vi "Stop Core.vi"(10 "final error code":i32, 11 "Caller in":refnum<class "Caller.lvclass">) -> (3 "Caller out":refnum<class "Caller.lvclass">)   [LabVIEW 2020, in "Caller.lvlib" / "Caller.lvclass"]
doc: "(<B>Filename</B>: Actor Framework.lvlib:Actor.lvclass:Stop Core.vi)\n\nDefines what the actor does before it stops. Use the <B>final error code</B> input to determine whether the actor shut down in response to an error.\n\nBy default, this method passes the Stop message along to all auto-stop nested actors. A descendant class may override this method to define additional behavior, such as shutting down any processes the actor initiated in its override of the Actor Core method."
uses:
  Caller.lvclass
  Caller.lvclass/Caller.ctl
  <vilib>/ActorFramework/Actor/Actor.lvclass
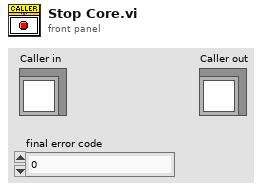
[diagram p1: front panel]
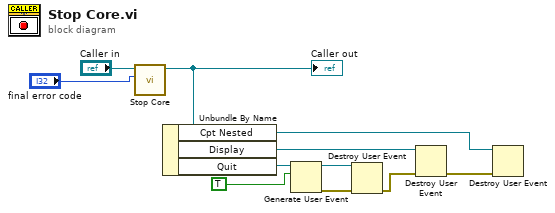
[diagram p0: block diagram]
diagram:
  n1 = call-parent "Stop Core.vi"("final error code"="final error code", "Actor in"="Caller in") -> ("Actor out"=w9:refnum<class "Caller.lvclass">)  [unwired: 9 in]
  "Caller out" <- w9
  n2 = Unbundle By Name(w9) -> ("Cpt Nested"=w1:refnum<user-event>, "Display"=w3:refnum<user-event>, "Quit"=w8:refnum<user-event>)
  n3 = Generate User Event(user event=w8, event data cluster=TRUE) -> (user event out=w6:refnum<user-event>, error out=w5:errorcluster)  [unwired: 2 in]
  n4 = Destroy User Event(user event=w6, error in=w5) -> (error out=w4:errorcluster)
  n5 = Destroy User Event(user event=w3, error in=w4) -> (error out=w2:errorcluster)
  n6 = Destroy User Event(user event=w1, error in=w2) -> ()  [unwired: 1 out]
